vi "Get File Path.vi"(8 "error in (no error)":errorcluster, 11 "DSF Configuration Reference in":T1) -> (0 "error out":errorcluster, 2 "file path":path, 3 "DSF Configuration Reference out":T1, 5 "need update":bool)   [LabVIEW 2017, in "DSF Core.lvlib" / "Configuration Session.lvclass"]
uses:
  Configuration Session.lvclass
  DSF Config Data Ref.ctl
  DSF Config Data.ctl
  Internal DSF Configuration.ctl
  Typedefs/DSF Version Info.ctl
  Internal DSF Plugin with ID.ctl
  Internal DSF Plugin Info.ctl
  Typedefs/DSF Timing Info.ctl
  Typedefs/DSF Engine Plugin Thread Configuration.ctl
  Typedefs/DSF Settings Info.ctl
  Internal DSF Group with ID.ctl
  Internal DSF Group Info.ctl
  Internal DSF Transfer with ID.ctl
  Internal DSF Transfer Info.ctl
  Internal DSF Channel with ID.ctl
  Internal DSF Channel Info.ctl
  Internal DSF Settings with ID.ctl
  Internal DSF Settings Info.ctl
  DSF Core.lvlib
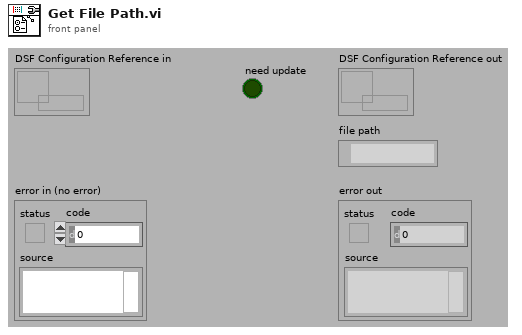
[diagram p1: front panel]
types:
  T1 = typedef "DSF Core.lvlib/Configuration Session.lvclass/DSF Config Data Ref.ctl" = refnum<data-value>
  T2 = typedef "DSF Core.lvlib/Configuration Session.lvclass/DSF Config Data.ctl" = cluster{"dsf configuration":T3, "path":path, "dirty":bool}
  T3 = typedef "DSF Core.lvlib/Configuration Session.lvclass/Internal DSF Configuration.ctl" = cluster{"dsfversion":T4, "version":T4, "plugins":T5[], "groups":T10[], "transfers":T12[], "channels":T14[], "settings":T16[]}
  T4 = typedef "DSF Core.lvlib/DSF Version Info.ctl" = cluster{"major":u32, "minor":u32, "fix":u32, "build":string}
  T5 = typedef "DSF Core.lvlib/Configuration Session.lvclass/Internal DSF Plugin with ID.ctl" = cluster{"id":string, "values":T6}
  T6 = typedef "DSF Core.lvlib/Configuration Session.lvclass/Internal DSF Plugin Info.ctl" = cluster{"components":string[], "timing":T7, "group ids":string[], "settings id":string, "threads":T8[]}
  T7 = typedef "DSF Core.lvlib/DSF Timing Info.ctl" = cluster{"priority":u64, "decimation":u64, "offset":u64}
  T8 = typedef "DSF Core.lvlib/DSF Engine Plugin Thread Configuration.ctl" = cluster{"buffer converter settings":T9, "transceiver settings":T9, "processor":i32, "priority offset":i16}
  T9 = typedef "DSF Core.lvlib/DSF Settings Info.ctl" = cluster{"key":string, "value":string}[]
  T10 = typedef "DSF Core.lvlib/Configuration Session.lvclass/Internal DSF Group with ID.ctl" = cluster{"id":string, "values":T11}
  T11 = typedef "DSF Core.lvlib/Configuration Session.lvclass/Internal DSF Group Info.ctl" = cluster{"direction":i32, "timing":T7, "transfer ids":string[], "settings id":string, "thread":i32, "timeout behavior":u8}
  T12 = typedef "DSF Core.lvlib/Configuration Session.lvclass/Internal DSF Transfer with ID.ctl" = cluster{"id":string, "values":T13}
  T13 = typedef "DSF Core.lvlib/Configuration Session.lvclass/Internal DSF Transfer Info.ctl" = cluster{"byte order":i32, "channel ids":string[], "settings id":string}
  T14 = typedef "DSF Core.lvlib/Configuration Session.lvclass/Internal DSF Channel with ID.ctl" = cluster{"id":string, "values":T15}
  T15 = typedef "DSF Core.lvlib/Configuration Session.lvclass/Internal DSF Channel Info.ctl" = cluster{"string buffer offset":u64, "string data type":i32, "engine data type":i32, "settings id":string}
  T16 = typedef "DSF Core.lvlib/Configuration Session.lvclass/Internal DSF Settings with ID.ctl" = cluster{"id":string, "values":T17}
  T17 = typedef "DSF Core.lvlib/Configuration Session.lvclass/Internal DSF Settings Info.ctl" = cluster{"key":string, "value":string}[]
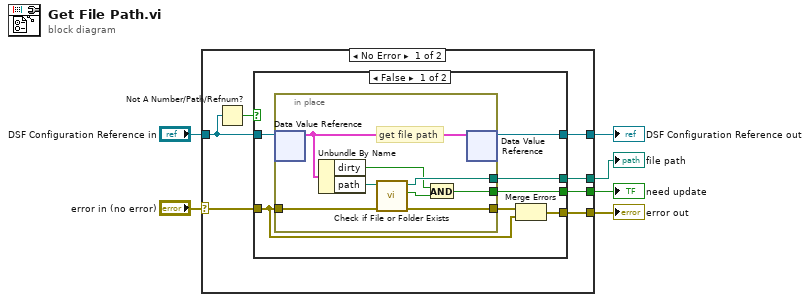
[diagram p0: block diagram]
diagram:
  n1 = case shown="No Error" "error in (no error)" {
    selector: "error in (no error)" -> [w10 w31]
    tunnel: "DSF Configuration Reference in" -> [w8 w32]
    tunnel: [w13 _] -> w6
    tunnel: [w11 w32] -> w2
    tunnel: [w12 w31] -> w4
    tunnel: [w9 _] -> w1
    frame No Error {
      n2 = Not A Number/Path/Refnum?(number/path/refnum=w8) -> (NaN/Path/Refnum?=w7:bool)
      n3 = case shown="False" w7 {
        tunnel: [w19 _] -> w13
        tunnel: [w16 w29] -> w12
        tunnel: w8 -> [w15 w30]
        tunnel: [w14 w30] -> w11
        tunnel: w10 -> [w20 w29]
        tunnel: [w18 _] -> w9
        frame False {
          n4 = in-place {
            in-place-border: w20 -> [w28]
            in-place-border: [w26] -> w19
            in-place-border: [w25] -> w18
            in-place-border: [w22] -> w17
            # "get file path"
            n5 = in-place-dvr #1(w15) -> (w21:T2)  [unwired: 1 out]
            n6 = Unbundle By Name(w21) -> ("dirty"=w24:bool, "path"=w27:path)
            n7 = call <vilib>:"Check if File or Folder Exists.vi"("error in (no error)"=w28, "path"=w27) -> ("error out"=w22:errorcluster, "file or folder exists?"=w23:bool, "dup path"=w26:path)  [unwired: 7 out]
            n8 = And(x=w24, y=w23) -> (x .and. y?=w25:bool)
            n9 = in-place-dvr #1(w21) -> (w14:T1)  [unwired: 1 out]
          }
          n10 = Merge Errors(w17, w20) -> (w16:errorcluster)
        }
        frame True {
        }
      }
    }
    frame Error {
    }
  }
  "error out" <- w4
  "file path" <- w6
  "DSF Configuration Reference out" <- w2
  "need update" <- w1
